vi "Data Update.vi"(0 "UpdatedDataIn":T1, 5 "OriginData":T1, 11 "error in (no error)":errorcluster) -> (4 "UpdateDataOut":T1, 15 "error out":errorcluster)   [LabVIEW 2018, in "Manipulate IPF.lvlib"]
uses:
  Manipulate IPF.lvlib
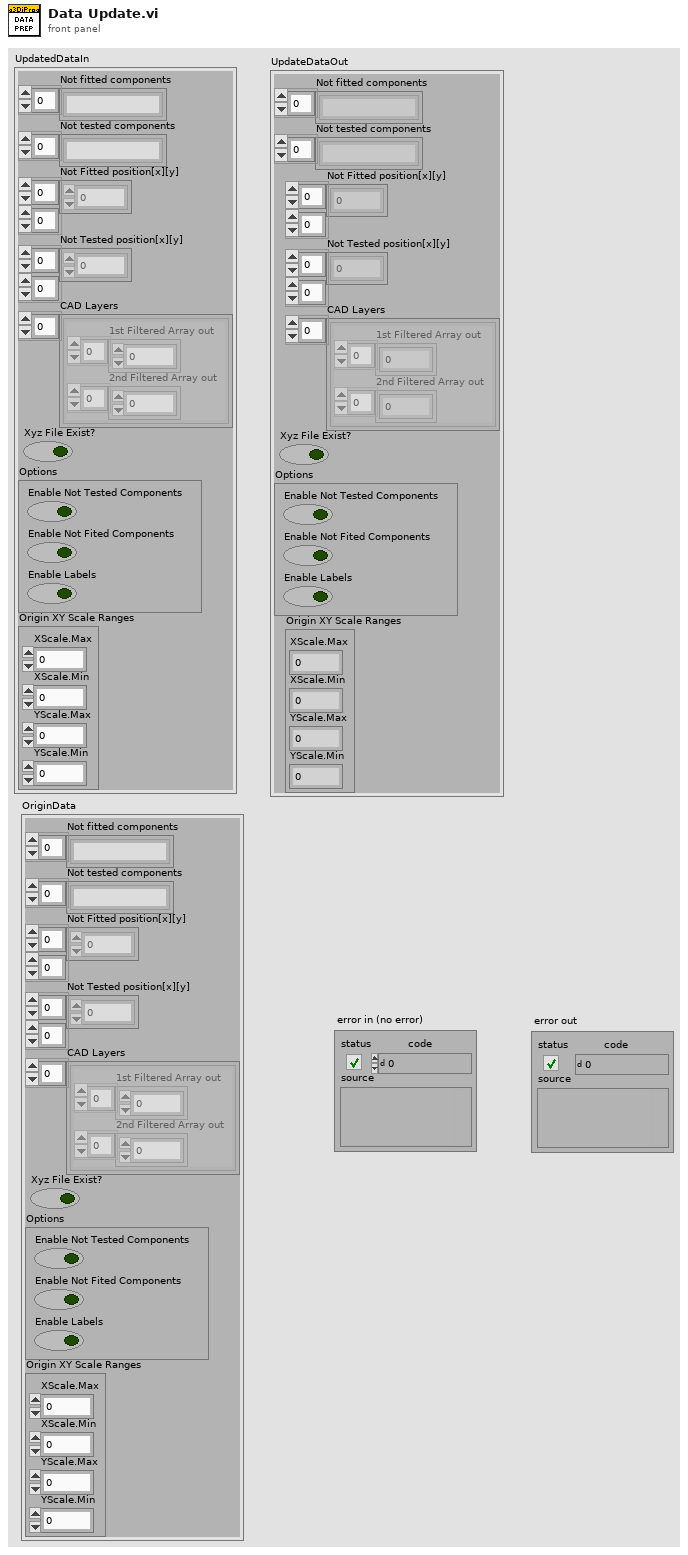
[diagram p1: front panel]
types:
  T1 = cluster{"Not fitted components":string[], "Not tested components":string[], "Not Fitted position[x][y] ":dbl[][], "Not Tested position[x][y]":dbl[][], "CAD Layers":cluster{"1st Filtered Array out":sgl[], "2nd Filtered Array out":sgl[]}[], "Xyz File Exist? ":bool, "Options":cluster{"Enable Not Tested Components":bool, "Enable Not Fited Components":bool, "Enable Labels":bool}, "Origin XY Scale Ranges":cluster{"XScale.Max":dbl, "XScale.Min":dbl, "YScale.Max":dbl, "YScale.Min":dbl}}
  T2 = cluster{"1st Filtered Array out":sgl[], "2nd Filtered Array out":sgl[]}
  T3 = cluster{"1st Filtered Array out":sgl[], "2nd Filtered Array out":sgl[]}[]
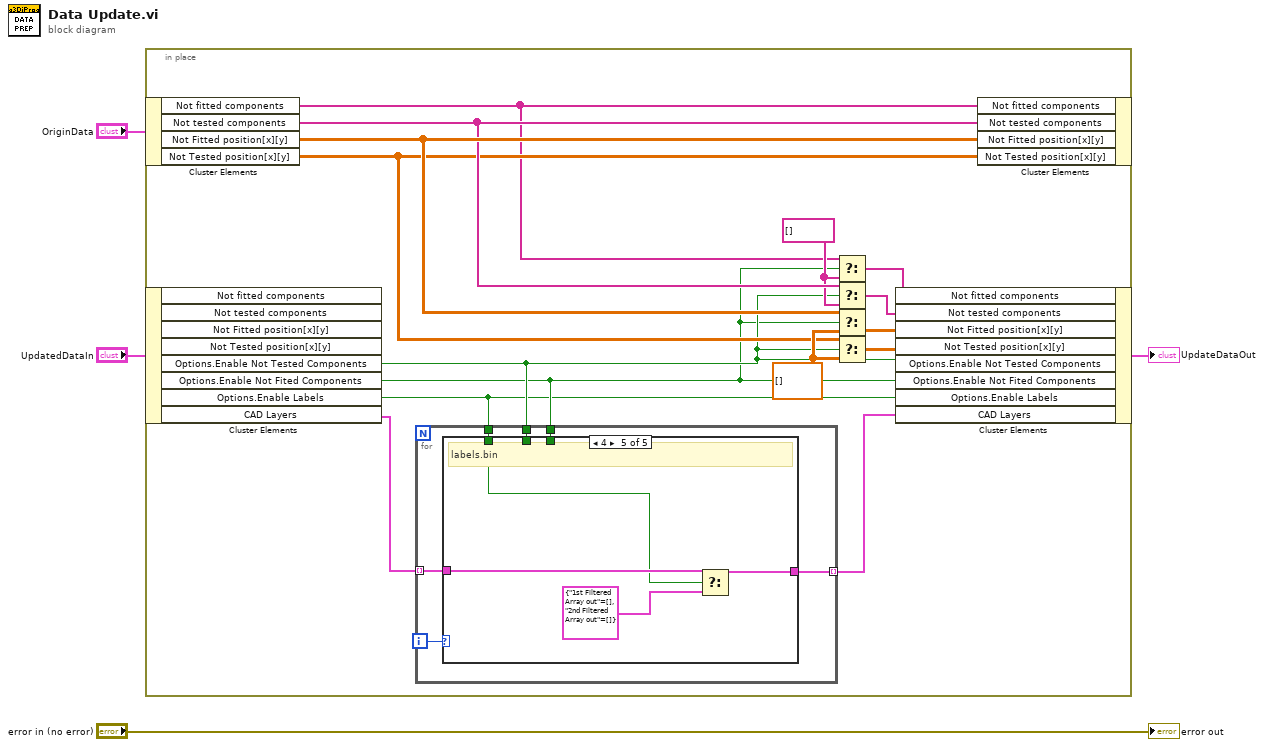
[diagram p0: block diagram]
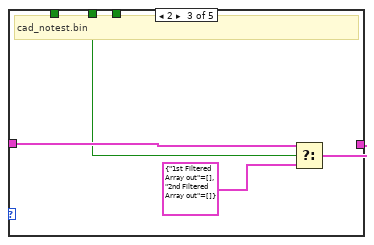
[diagram p4: hidden frame]
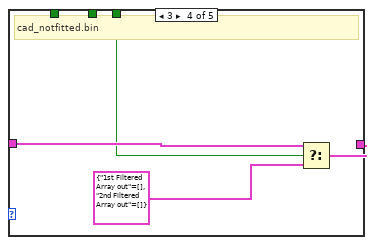
[diagram p5: hidden frame]
diagram:
  n1 = in-place {
    w12 = string[] [] ("f")
    w15 = dbl[][] [] ("f")
    n2 = in-place-cluster #1("OriginData") -> ("Not fitted components"=w10:string[], "Not tested components"=w13:string[], "Not Fitted position[x][y]"=w14:dbl[][], "Not Tested position[x][y]"=w11:dbl[][])
    n3 = in-place-cluster #2("UpdatedDataIn") -> ("Options.Enable Not Tested Components"=w7:bool, "Options.Enable Not Fited Components"=w6:bool, "Options.Enable Labels"=w5:bool, "CAD Layers"=w9:T3)  [unwired: 4 out]
    n4 = for {
      tunnel: w9 -> [w25] mode=indexing
      tunnel: [w23] -> w8 mode=indexing
      tunnel: w7 -> [w22]
      tunnel: w6 -> [w21]
      tunnel: w5 -> [w20]
      i -> [w24]
      n5 = case shown="4" w24 {
        tunnel: w25 -> [w26 w27 w31 w35 w39]
        tunnel: [w26 w27 w30 w34 w38] -> w23
        tunnel: w22 -> [_ _ w28 _ _]
        tunnel: w21 -> [_ _ _ w32 _]
        tunnel: w20 -> [_ _ _ _ w36]
        frame 0, Default {
          # "XYZ layer"
        }
        frame 1 {
          # "cad_tested.bin"
        }
        frame 2 {
          # "cad_notest.bin"
          n6 = Select(t=w31, s=w28, f=T2 {"1st Filtered Array out"=[], "2nd Filtered Array out"=[]}) -> (s? t:f=w30:T2)
        }
        frame 3 {
          # "cad_notfitted.bin"
          n7 = Select(t=w35, s=w32, f=T2 {"1st Filtered Array out"=[], "2nd Filtered Array out"=[]}) -> (s? t:f=w34:T2)
        }
        frame 4 {
          # "labels.bin"
          n8 = Select(t=w39, s=w36, f=T2 {"1st Filtered Array out"=[], "2nd Filtered Array out"=[]}) -> (s? t:f=w38:T2)
        }
      }
    }
    n9 = Select(t=w10, s=w6, f=w12) -> (s? t:f=w19:string[])
    n10 = Select(t=w13, s=w7, f=w12) -> (s? t:f=w18:string[])
    n11 = Select(t=w14, s=w6, f=w15) -> (s? t:f=w17:dbl[][])
    n12 = Select(t=w11, s=w7, f=w15) -> (s? t:f=w16:dbl[][])
    n13 = in-place-cluster #2("Not fitted components"=w19, "Not tested components"=w18, "Not Fitted position[x][y]"=w17, "Not Tested position[x][y]"=w16, "Options.Enable Not Tested Components"=w7, "Options.Enable Not Fited Components"=w6, "Options.Enable Labels"=w5, "CAD Layers"=w8) -> (→"UpdateDataOut":T1)
    n14 = in-place-cluster #1("Not fitted components"=w10, "Not tested components"=w13, "Not Fitted position[x][y]"=w14, "Not Tested position[x][y]"=w11) -> ()  [unwired: 1 out]
  }
  "error out" <- "error in (no error)"
